vi "niScope EX Multi Record Fetch More Than Available Memory Producer Consumer 8_6.vi"() -> ()   [LabVIEW 2009]
doc: "Example: Multi Record Fetch More Than Available Memory\n\nRecommended Input Signal: 1 kHz, 1.8 Vpp, sine wave\n\nDevices Supported: Refer to NI Example Finders\n\nLabVIEW Description:\n\nThis VI demonstrates the multi-record and continuous acquisition capabilities of National Instruments digitizers. In a multi-record acquisition, each record is one waveform with at least \"min record length\" points as specified with the Configure Horizontal Timing VI. Furthermore, each record is triggered, so when the trigger arrives for the first record, the hardware quickly rearms for the next record. Refer the to Multi Record example for more information.\n\nIn this example, the Fetch VI is used with the Fetch Record Number and Fetch Number of Records properties to fetch each record individually. Using the Fetch VI with a positive timeout only waits for the requested waveform to be done - rather than waiting for all the records. In this example, the fetch VI only waits for the next record, and than it retrieves the record while it is acquiring other records. \n\nThe Allow More Records Than Memory property is a Boolean value that allows you to configure more records than fit in the onboard memory at one time. When this is enabled, you can specify any number of records. The records are treated circularly in the onboard memory, so you must fetch them before they are overwritten. If you attempt to fetch a record that has been overwritten in the digitizer's memory, an error is returned. \n\nWarning! Windows NT and 2000 limit the amount of page locked memory at any given time, and they will crash without warning if you exceed this limit. Every record that you configure requires a small amount of page locked memory, so be careful when configuring a large number of records! \n\nSee the NI High Speed Digitizers Help for more information about continuous, multiple-record acquisitions.\n\nThis example allows you to disable plotting. Fetching will be much faster if plotting is not enabled. If it is enabled, the last record fetched will be displayed on the graph."
uses:
  <instrlib>/niScope/Controls/niScope trigger slope.ctl
  <instrlib>/niScope/Controls/niScope trigger coupling.ctl
  <instrlib>/niScope/Controls/niScope trigger source.ctl
  <instrlib>/niScope/Configure/Trigger/niScope Configure Trigger Edge.vi
  <instrlib>/niScope/Acquire/Fetch/niScope Multi Fetch WDT.vi
panel:
  out "error out":errorcluster {"code" format="%.0x"}
  in  "stop":bool
  in  "edge trigger level":dbl format="%.2f"
  in  "Allow more records\nthan available memory?":bool=TRUE
  out "# Acquired":i32=100 caption="Number of Records Acquired"
  in  "number of records":i32=100 caption="Number of Records"
  in  "channel name":string="0"
  in  "Plot Data?":bool=TRUE
  in  "resource name":refnum<k15>="DAQ::1"
  out "# Fetched":i32=100 caption="Number of Records Fetched"
  in  "min record length":i32=8192
  out "Last Record Fetched":waveform(dbl)[](graph)
  in  "min sample rate":dbl=10000000.0 step=1000000.0 format="%.3p"
  in  "vertical range":dbl=2.0 format="%.2f"
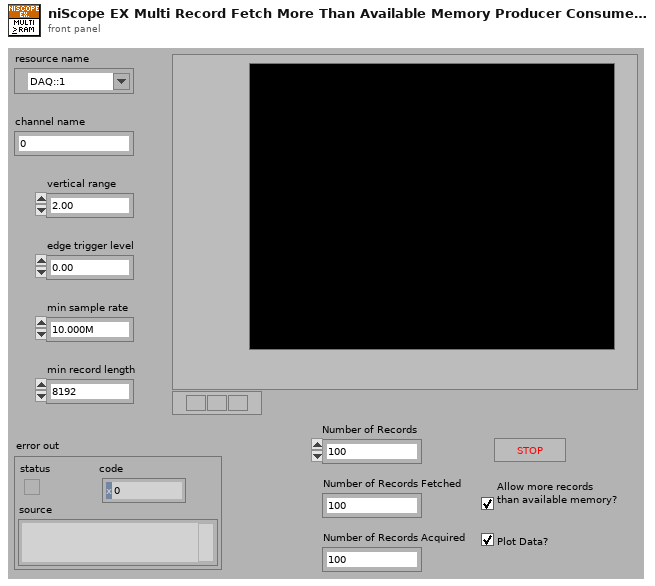
[diagram p1: front panel]
types:
  T1 = enum16{"open", "open or create", "create or replace", "create", "open (read-only)"}
  T2 = typedef "niScope trigger source.ctl" = string
  T3 = typedef "niScope trigger coupling.ctl" = u16
  T4 = typedef "niScope trigger slope.ctl" = i32
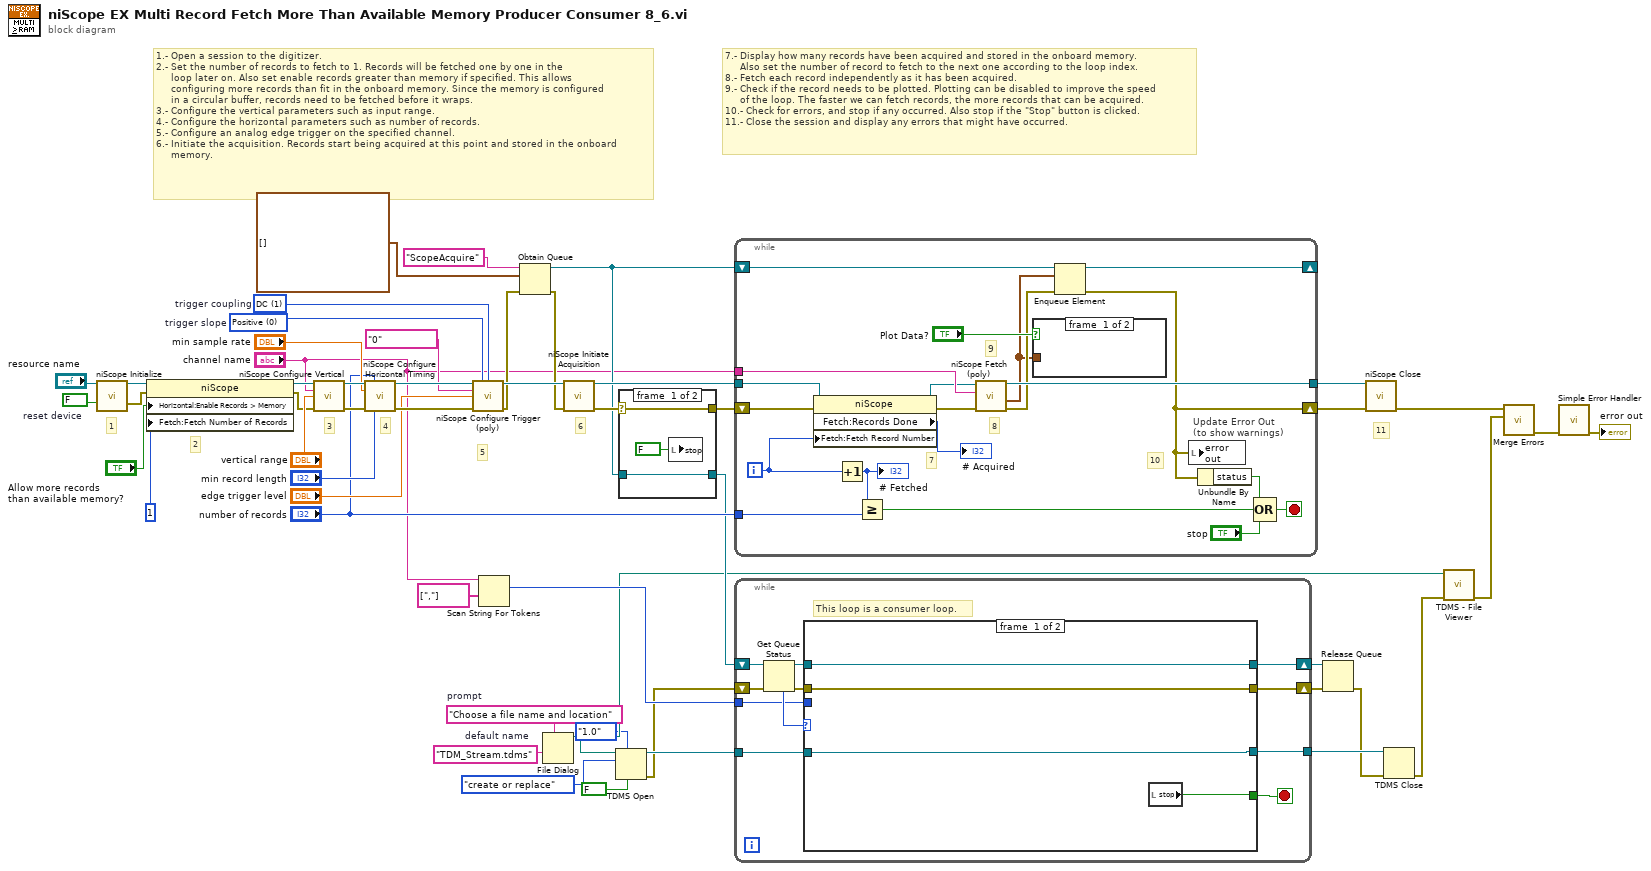
[diagram p0: block diagram]
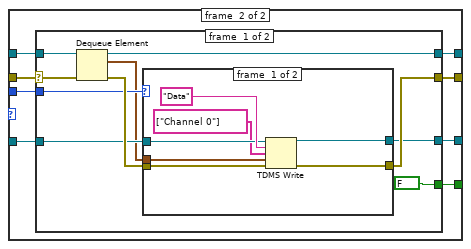
[diagram p3: hidden frame]
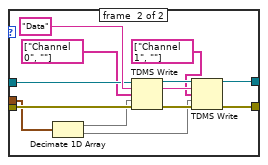
[diagram p4: hidden frame]
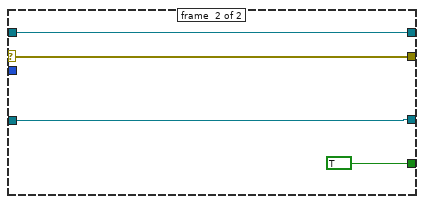
[diagram p5: hidden frame]
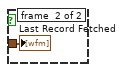
[diagram p6: hidden frame]
diagram:
  w16 = "TDM_Stream.tdms"  # default name
  w15 = "Choose a file name and location"  # prompt
  w32 = T3 1 items=["AC"=0, "DC"=1, "HF Reject"=3, "LF Reject"=4, "AC Plus HF Reject"=1001]  # trigger coupling
  w33 = T4 0 items=["Positive", "Negative"]  # trigger slope
  w52 = FALSE  # reset device
  # "7.- Display how many records have been acquired and stored in the onboard memory.\n     Also set the number of record to fetch to the next one according to the loop index.\n8.- Fetch each record independently as it has been acquired.\n9.- Check if the record needs to be plotted. Plotting can be disabled to improve the speed\n     of the loop. The faster we can fetch records, the more records that can be acquired.\n10.- Check for errors, and stop if any occurred. Also stop if the \"Stop\" button is clicked.\n11.- Close the session and display any errors that might have occurred."
  # "1.- Open a session to the digitizer.\n2.- Set the number of records to fetch to 1. Records will be fetched one by one in the\n     loop later on. Also set enable records greater than memory if specified. This allows\n     configuring more records than fit in the onboard memory. Since the memory is configured\n     in a circular buffer, records need to be fetched before it wraps.\n3.- Configure the vertical parameters such as input range.\n4.- Configure the horizontal parameters such as number of records.\n5.- Configure an analog edge trigger on the specified channel. \n6.- Initiate the acquisition. Records start being acquired at this point and stored in the onboard\n     memory."
  # "11"
  # "6"
  # "5"
  # "4"
  # "3"
  # "2"
  # "1"
  n1 = call <instrlib>:"niScope Initialize.vi"("resource name"="resource name", "reset device"=w52) -> ("instrument handle"=w49:refnum<k15>, "error out"=w48:errorcluster)  [unwired: 2 in, 10 out]
  n2 = property class="niScope"(reference=w49, error in=w48, "Horizontal:Enable Records > Memory"="Allow more records\nthan available memory?", "Fetch:Fetch Number of Records"=1) -> (reference out=w47:refnum<k15>, error out=w46:errorcluster)
  n3 = call <instrlib>:"niScope Configure Vertical.vi"("instrument handle"=w47, "channels"="channel name", "vertical range"="vertical range", "error in"=w46) -> ("instrument handle out"=w44:refnum<k15>, "error out"=w43:errorcluster)  [unwired: 4 in, 6 out]
  n4 = call <instrlib>:"niScope Configure Horizontal Timing.vi"("instrument handle"=w44, "number of records"="number of records", "min sample rate"="min sample rate", "error in"=w43, "min record length"="min record length") -> ("instrument handle out"=w40:refnum<k15>, "error out"=w38:errorcluster)  [unwired: 2 in, 7 out]
  n5 = call-poly <instrlib>:"niScope Configure Trigger (poly).vi"("instrument handle"=w40, "trigger slope"=w33, "trigger coupling"=w32, "trigger source"=T2 "0", "trigger level"="edge trigger level", "error in"=w38) -> ("instrument handle out"=w39:refnum<k15>, "error out"=w26:errorcluster)  [unwired: 2 in, 6 out]
  n6 = Scan String For Tokens(7:string[] [","] ("operators (none)"), 9:"channel name") -> (2:w12:i32)  [unwired: 1 in, 6 out]
  n7 = Obtain Queue(name (unnamed)="ScopeAcquire", element data type=waveform(dbl)[] [] ("wfm"), error in (no error)=w26) -> (queue out=w22:refnum<queue>, error out=w27:errorcluster)  [unwired: 2 in, 1 out]
  n8 = File Dialog(7:w15, 9:w16) -> (3:w9:path)  [unwired: 1 in, 7 out]
  n9 = call <instrlib>:"niScope Initiate Acquisition.vi"("instrument handle"=w39, "error in"=w27) -> ("instrument handle out"=w31:refnum<k15>, "error out"=w23:errorcluster)  [unwired: 12 out]
  n10 = TDMS Open(6:FALSE ("disable buffering (T)"), 7:enum16{"1.0", "2.0"}."1.0" ("file format version (2.0)"), 10:T1."create or replace" ("operation"), 11:w9) -> (0:w10:errorcluster, 3:w11:refnum<k34>)  [unwired: 2 in]
  n11 = case shown="No Error" w23 {
    selector: w23 -> [w53 w57]
    tunnel: w22 -> [w54 w56]
    tunnel: [w54 w56] -> w21
    tunnel: [w53 w57] -> w20
    frame #0 {
      n12 = local write "stop"(FALSE ("stop")) -> ()
    }
    frame #1 {
    }
  }
  n13 = while {
    tunnel: "number of records" -> [w77]
    tunnel: "channel name" -> [w74]
    tunnel: w31 -> [w65]
    tunnel: [w63] -> w29
    shift-right: [w59] -> _
    shift-left: w22 -> [w62]
    shift-right: [w60] -> w30
    shift-left: w20 -> [w64]
    i -> [w71]
    stop <- w76 stop-if-true
    # "10"
    # "9"
    # "8"
    # "7"
    # "Update Error Out\n(to show warnings)"
    n14 = property class="niScope"(reference=w65, error in=w64, "Fetch:Fetch Record Number"=w71) -> (reference out=w66:refnum<k15>, error out=w70:errorcluster, "Fetch:Records Done"=→"# Acquired":i32)
    n15 = Increment(x=w71) -> (x+1=w73:i32)
    "# Fetched" <- w73
    n16 = Greater Or Equal?(x=w73, y=w77) -> (x >= y?=w69:bool)
    n17 = call-poly <instrlib>:"niScope Fetch (poly).vi"("error in"=w70, "channels"=w74, "instrument handle"=w66) -> ("error out"=w61:errorcluster, "wfm"=w58:waveform(dbl)[], "instrument handle out"=w63:refnum<k15>)  [unwired: 3 in, 3 out]
    n18 = case shown="True" "Plot Data?" {
      tunnel: w58 -> [_ w78]
      frame #0 {
      }
      frame #1 {
        "Last Record Fetched" <- w78
      }
    }
    n19 = Enqueue Element(queue=w62, element=w58, error in (no error)=w61) -> (queue out=w59:refnum<queue>, error out=w60:errorcluster)  [unwired: 2 out]
    n20 = local write "error out"(w60) -> ()
    n21 = Unbundle By Name(w60) -> ("status"=w68:bool)
    n22 = Compound Arithmetic op=OR(w68, w69, "stop") -> (w76:bool)
  }
  n23 = while {
    shift-right: [w84] -> w19
    shift-left: w21 -> [w88]
    shift-right: [w83] -> w18
    shift-left: w10 -> [w82]
    tunnel: w12 -> [w80]
    tunnel: w11 -> [w81]
    tunnel: [w79] -> w8
    stop <- w89 stop-if-true
    # "This loop is a consumer loop."
    n24 = Get Queue Status(queue=w88, error in (no error)=w82) -> (queue out=w85:refnum<queue>, error out=w87:errorcluster, # elements in queue=w86:i32)  [unwired: 6 out]
    n25 = case shown="0" w86 {
      tunnel: [w93 w100] -> w89
      tunnel: w87 -> [w91 w101]
      tunnel: w85 -> [w90 w99]
      tunnel: [w90 w98] -> w84
      tunnel: [w91 w97] -> w83
      tunnel: w81 -> [w92 w96]
      tunnel: w80 -> [_ w95]
      tunnel: [w92 w94] -> w79
      frame #0 {
        n26 = local read "stop"() -> (w93:bool)
      }
      frame #1 {
        n27 = case shown="No Error" w101 {
          selector: w101 -> [w109 w133]
          tunnel: [FALSE TRUE] -> w100
          tunnel: w99 -> [w110 w132]
          tunnel: [w108 w132] -> w98
          tunnel: [w105 w133] -> w97
          tunnel: w96 -> [w106 w134]
          tunnel: w95 -> [w104 _]
          tunnel: [w102 w134] -> w94
          frame #0 {
            n28 = Dequeue Element(queue=w110, error in (no error)=w109) -> (queue out=w108:refnum<queue>, element=w103:waveform(dbl)[], error out=w107:errorcluster)  [unwired: 2 out]
            n29 = case shown="0, Default" w104 {
              tunnel: w107 -> [w117 w130]
              tunnel: w106 -> [w116 w129]
              tunnel: [w112 w119] -> w105
              tunnel: w103 -> [w114 w127]
              tunnel: [w113 w120] -> w102
              frame #0 {
                n30 = TDMS Write(0:w116, 5:"Data" ("group name in"), 7:string[] ["Channel 0"] ("channel name(s) in (Untitled)"), 9:w114, 11:w117) -> (4:w113:refnum<k34>, 15:w112:errorcluster)  [unwired: 1 in, 2 out]
              }
              frame #1 {
                n31 = Decimate 1D Array(w127) -> (w122:waveform(dbl)[], w121:waveform(dbl)[])
                n32 = TDMS Write(0:w129, 5:"Data" ("group name in"), 7:string[] ["Channel 0", ""] ("channel name(s) in (Untitled)"), 9:w122, 11:w130) -> (4:w126:refnum<k34>, 6:w125:string, 15:w124:errorcluster)  [unwired: 1 in, 1 out]
                n33 = TDMS Write(0:w126, 5:w125, 7:string[] ["Channel 1", ""] ("channel name(s) in (Untitled)"), 9:w121, 11:w124) -> (4:w120:refnum<k34>, 15:w119:errorcluster)  [unwired: 1 in, 2 out]
              }
            }
          }
          frame #1 {
          }
        }
      }
    }
  }
  n34 = Release Queue(queue=w19, error in (no error)=w18) -> (error out=w7:errorcluster)  [unwired: 3 out]
  n35 = call <instrlib>:"niScope Close.vi"("instrument handle"=w29, "error in"=w30) -> ("error out"=w4:errorcluster)  [unwired: 13 out]
  n36 = TDMS Close(8:w7, 11:w8) -> (0:w6:errorcluster)
  n37 = call <vilib>:"TDMS - File Viewer.vi"("error in (no error)"=w6, "file path"=w9) -> ("error out"=w3:errorcluster)  [unwired: 5 out]
  n38 = call <vilib>:"Merge Errors.vi"("error in 2 (no error)"=w3, "error in 1 (no error)"=w4) -> ("error out"=w5:errorcluster)  [unwired: 2 in, 3 out]
  n39 = call <vilib>:"Simple Error Handler.vi"("error in (no error)"=w5) -> ("error out"=→"error out":errorcluster)  [unwired: 1 in, 7 out]
